vi "EPS-Device Information.vi"(8 "error in":errorcluster, 11 "EPS Setting In":T2) -> (0 "error out":errorcluster, 2 "Device Information":T1, 3 "EPS Setting Out":T2)   [LabVIEW 2018]
uses:
  Data Def/EPS-Setting.ctl
  Data Def/EPS-Access Mode.ctl
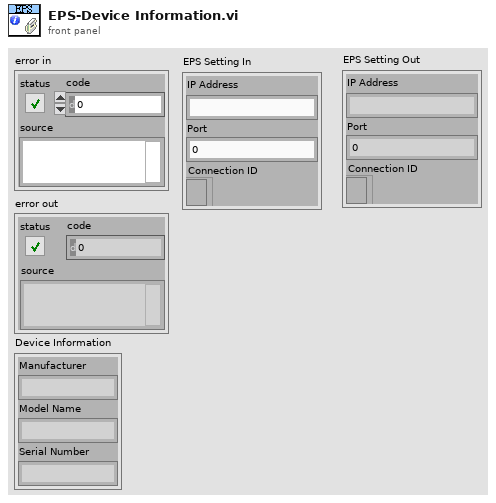
[diagram p1: front panel]
types:
  T1 = cluster{"Manufacturer":string, "Model Name":string, "Serial Number":string}
  T2 = typedef "EPS-Setting.ctl" = cluster{"IP Address":string, "Port":u16, "Connection ID":refnum<k5>}
  T3 = typedef "EPS-Access Mode.ctl" = enum16{"Read", "Write"}
  T4 = cluster{"String":string, "String":string, "String":string}
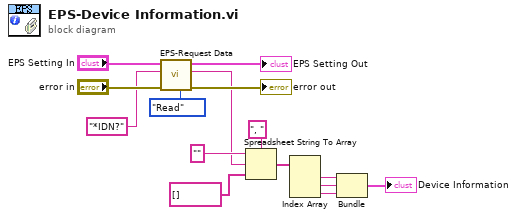
[diagram p0: block diagram]
diagram:
  n1 = call "EPS-Request Data.vi"("Access Mode"=EPS-Access_Mode."Read", "error in"="error in", "Requst Data"="*IDN?", "EPS Setting In"="EPS Setting In") -> ("error out"=→"error out":errorcluster, "Response Data"=w6:string, "EPS Setting Out"=→"EPS Setting Out":T2)  [unwired: 5 in]
  n2 = Spreadsheet String To Array(delimiter (Tab)=", ", format string="", spreadsheet string=w6, array type (2D Dbl)=string[] []) -> (array=w5:string[])
  n3 = Index Array(array=w5) -> (element #1=w4:string, element #2=w3:string, element #3=w2:string)  [unwired: 3 in]
  n4 = Bundle("String"=w4, "String"=w3, "String"=w2) -> (→"Device Information":T4)  [unwired: 1 in]
